vi "AlarmDeltas.vi"(0 "TimeStamp in":dbl[](array[numeric]), 5 "AlarmArray":dbl[][](array[numeric]), 7 "ChannelNames":string[](array[string])=["AI 0", "AI 1", "AI 2", "TC 0", "TC 1", "TC 2", "Temp 1"]) -> (4 "TimeStamp out":dbl[](array[numeric]), 8 "DeltasFound":i32, 10 "AlarmDeltaArray":dbl[][](array[numeric]), 15 "Alarm List":string[][](table))   [LabVIEW 2018]
doc: "Given the full time array of alarm data, scan through to find only the points in time where there are changes. Output an array of timestamps and corresponding data where these changes occur.\n\nAlarmDeltaArray stores the previous iteration data and current iteration data where any changes occured. \n\nAlarm List is a table of strings where each row is an Alarm with associated timestamp, channel number, and channel name."
panel:
  # "Previous                                                                                                                                           Current"
  # "0       1        2       3        4         5        6        7         8       9        10       11     12      13      14      0       1        2       3        4         5        6        7         8       9        10       11     12      13      14"
  # "Time"
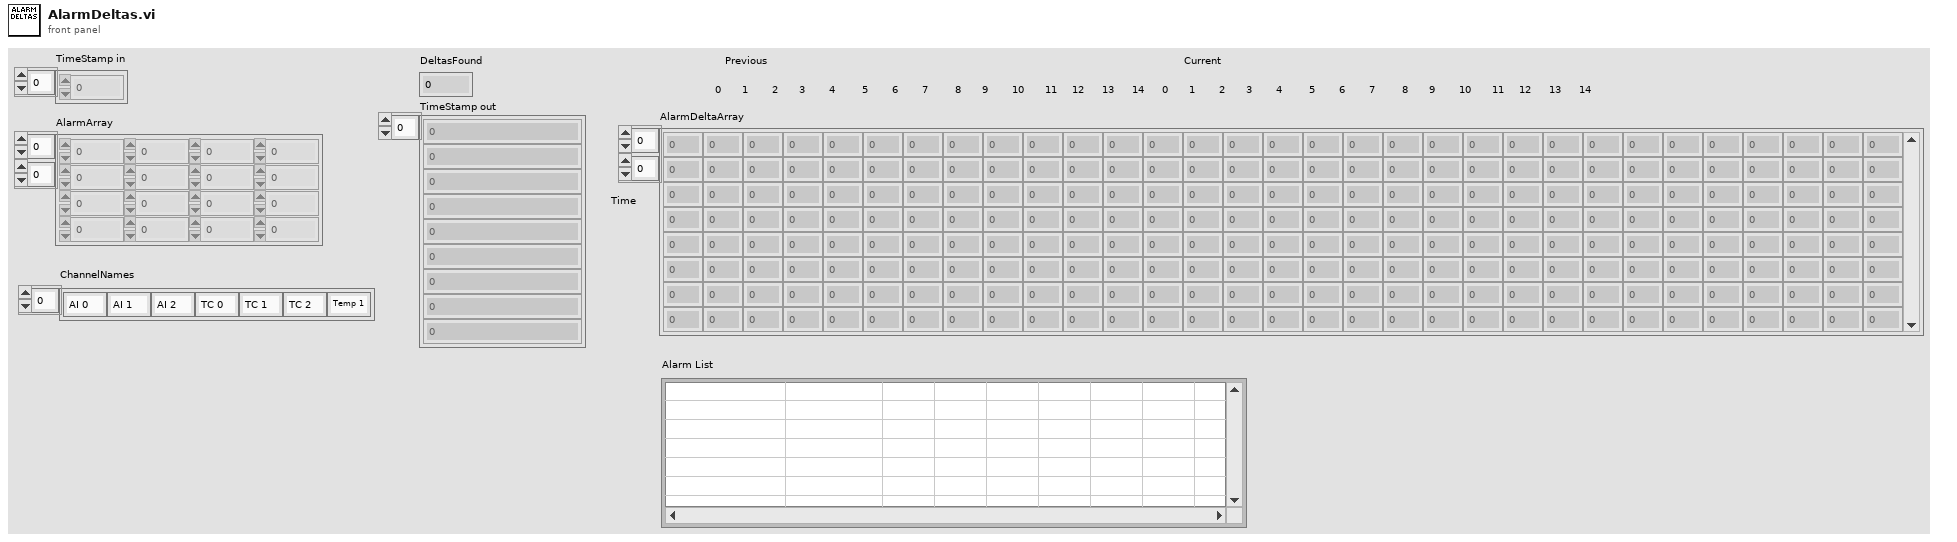
[diagram p1: front panel]
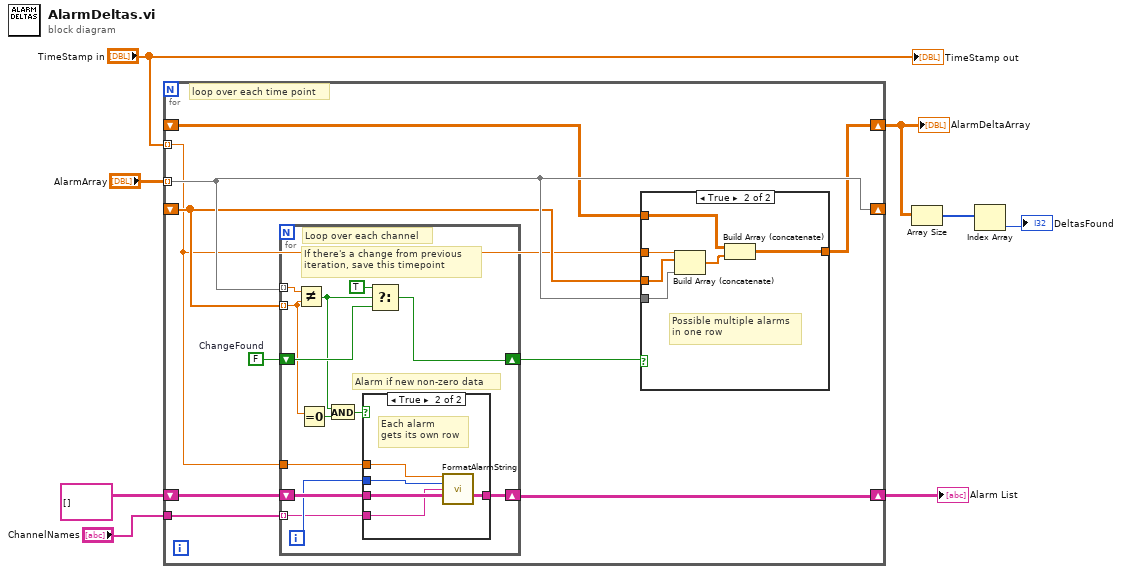
[diagram p0: block diagram]
diagram:
  n1 = for {
    tunnel: "AlarmArray" -> [w16] mode=indexing
    tunnel: "TimeStamp in" -> [w11] mode=indexing
    shift-right: [w16] -> _
    shift-left: _ -> [w15]
    shift-right: [w14] -> w6
    shift-left: _ -> [w13]
    shift-right: [w10] -> w2
    shift-left: string[][] [] ("Table Control") -> [w12]
    tunnel: "ChannelNames" -> [w9]
    w18 = FALSE  # ChangeFound
    # "loop over each time point"
    n2 = for {
      tunnel: w16 -> [w38] mode=indexing
      shift-right: [w36] -> w17
      shift-left: w18 -> [w37]
      tunnel: w15 -> [w26] mode=indexing
      tunnel: w11 -> [w34]
      shift-right: [w30] -> w10
      shift-left: w12 -> [w32]
      tunnel: w9 -> [w29] mode=indexing
      i -> [w31]
      # "Alarm if new non-zero data"
      # "If there's a change from previous \niteration, save this timepoint"
      # "Loop over each channel"
      n3 = Not Equal?(x=w38, y=w26) -> (x != y?=w33:bool)
      n4 = Equal To 0?(x=w26) -> (x = 0?=w27:bool)
      n5 = And(x=w33, y=w27) -> (x .and. y?=w28:bool)
      n6 = case shown="True" w28 {
        tunnel: w34 -> [_ w44]
        tunnel: w32 -> [w39 w42]
        tunnel: w31 -> [_ w43]
        tunnel: [w39 w41] -> w30
        tunnel: w29 -> [_ w40]
        frame False {
        }
        frame True {
          # "Each alarm\ngets its own row"
          n7 = call "FormatAlarmString.vi"("Timestamp_sec"=w44, "ChannelIndex"=w43, "ChannelName"=w40, "AlarmTableIn"=w42) -> ("AlarmTableOut"=w41:string[][])  [unwired: 11 in]
        }
      }
      n8 = Select(t=TRUE, s=w33, f=w37) -> (s? t:f=w36:bool)
    }
    n9 = case shown="True" w17 {
      tunnel: w11 -> [_ w25]
      tunnel: w16 -> [_ w23]
      tunnel: w15 -> [_ w24]
      tunnel: [w19 w21] -> w14
      tunnel: w13 -> [w19 w20]
      frame False {
      }
      frame True {
        # "Possible multiple alarms\nin one row"
        n10 = Build Array (concatenate)(w25, w24, w23) -> (w22:dbl[])
        n11 = Build Array (concatenate)(w20, w22) -> (w21:dbl[][])
      }
    }
  }
  "AlarmDeltaArray" <- w6
  "Alarm List" <- w2
  n12 = Array Size(array=w6) -> (size(s)=w5:i32[])
  n13 = Index Array(array=w5) -> (element=→"DeltasFound":i32)  [unwired: 1 in]
  "TimeStamp out" <- "TimeStamp in"
